vi "Calc Hash.vi"(11 "String":string) -> (3 "Numeric":i32)   [LabVIEW 2021]
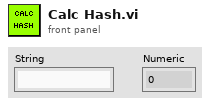
[diagram p1: front panel]
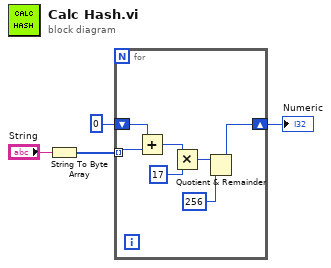
[diagram p0: block diagram]
diagram:
  n1 = String To Byte Array(string="String") -> (unsigned byte array=w2:u8[])
  n2 = for {
    tunnel: w2 -> [w11] mode=indexing
    shift-right: [w5] -> w4
    shift-left: 0 -> [w10]
    n3 = Add(x=w10, y=w11) -> (x+y=w9:i32)
    n4 = Multiply(x=w9, y=17) -> (x*y=w7:i32)
    n5 = Quotient & Remainder(x=w7, y=256) -> (x-y*floor(x/y)=w5:i32)  [unwired: 1 out]
  }
  "Numeric" <- w4
